vi "Worker Mode Status Example.vi"() -> ()   [LabVIEW 2017]
doc: "------------- lvcsm -------------\n[CSMStates]\nItem 0 = \"Event Structure\"\nItem 1 = \"Idle\"\nItem 2 = \"CSM Documentation\"\nItem 3 = \"VI Reference\"\nItem 4 = \"Error Handler\"\nItem 5 = \"Critical Error\"\nItem 6 = \"Target Busy Error\"\nItem 7 = \"Target Timeout Error\"\nItem 8 = \"Target Error\"\nItem 9 = \"Async Response\"\nItem 10 = \"Response\"\nItem 11 = \"Async Message Posted\"\nItem 12 = \"Initialize Core Data\"\nItem 13 = \"Exit\"\nItem 14 = \"Data: Initialize\"\nItem 15 = \"Data: Cleanup\"\nItem 16 = \"Events: Register\"\nItem 17 = \"Events: Unregister\"\nItem 18 = \"UI: Initialize\"\nItem 19 = \"UI: Cursor Set\"\nItem 20 = \"UI: Front Panel State\"\nItem 21 = \"Macro: Initialize\"\nItem 22 = \"Macro: Switch Active Module\"\nItem 23 = \"Macro: Exit\"\nItem 24 = \"Action: Status Chanage Handler\"\n\n[CSMStatus]"
uses:
  user.lib/_NEVSTOP/Communicable State Machine(CSM)/_Polymophic/Build Synchronous Message with Arguments.vi
  user.lib/_NEVSTOP/Communicable State Machine(CSM)/_Polymophic/Build No-Reply Asynchronous Message with Arguments.vi
  user.lib/_NEVSTOP/Communicable State Machine(CSM)/_Polymophic/Build Unregister Status Message.vi
  user.lib/_NEVSTOP/Communicable State Machine(CSM)/_Polymophic/Build Register Status Message.vi
  user.lib/_NEVSTOP/Communicable State Machine(CSM)/Communicable State Machine.lvlib
  examples/NEVSTOP/Communicable State Machine(CSM)/1. Create a reuse Module/1. Create a reuse Module.lvlib
panel:
  in  "UI: Front Panel State >> Close":bool
  in  "UI: Front Panel State >> Open":bool
  in  "Unregister All Status Change":bool
  in  "API: Stop":bool
  in  "API: Start":bool
  in  "Register All Status Change":bool
  out "State History of Main":string
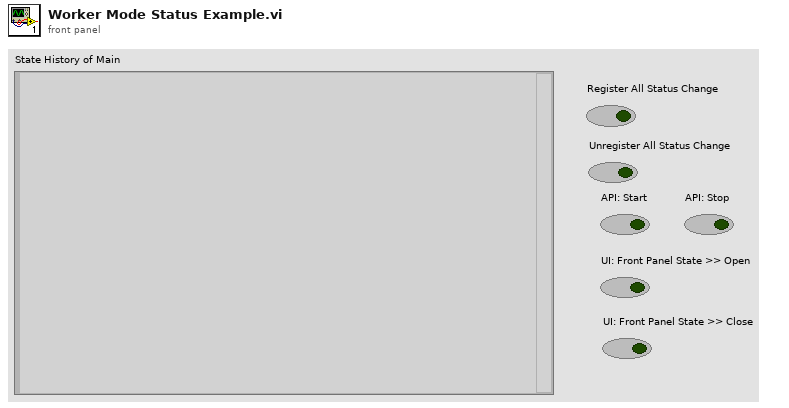
[diagram p1: front panel]
types:
  T1 = enum32{"Invalid", "Standard", "Closed", "Hidden", "Minimized", "Maximized"}
  T2 = enum32{"invalid app kind", "Development System", "Run Time System", "Student Edition", "Embedded LabVIEW", "Evaluation", "Custom"}
  T3 = typedef "Communicable State Machine.lvlib/_CSM_Response Source Message.ctl" = cluster{"‘State":string, "’Arguments":string, "’Error":errorcluster}
  T4 = cluster{"Current VI Reference":refnum<vi>, "Close Panel on Exit?":bool}
  T5 = cluster{"Core":cluster{"Current VI Reference":refnum<vi>, "Close Panel on Exit?":bool}, "Your Boolean data":bool, "Your string data":string}
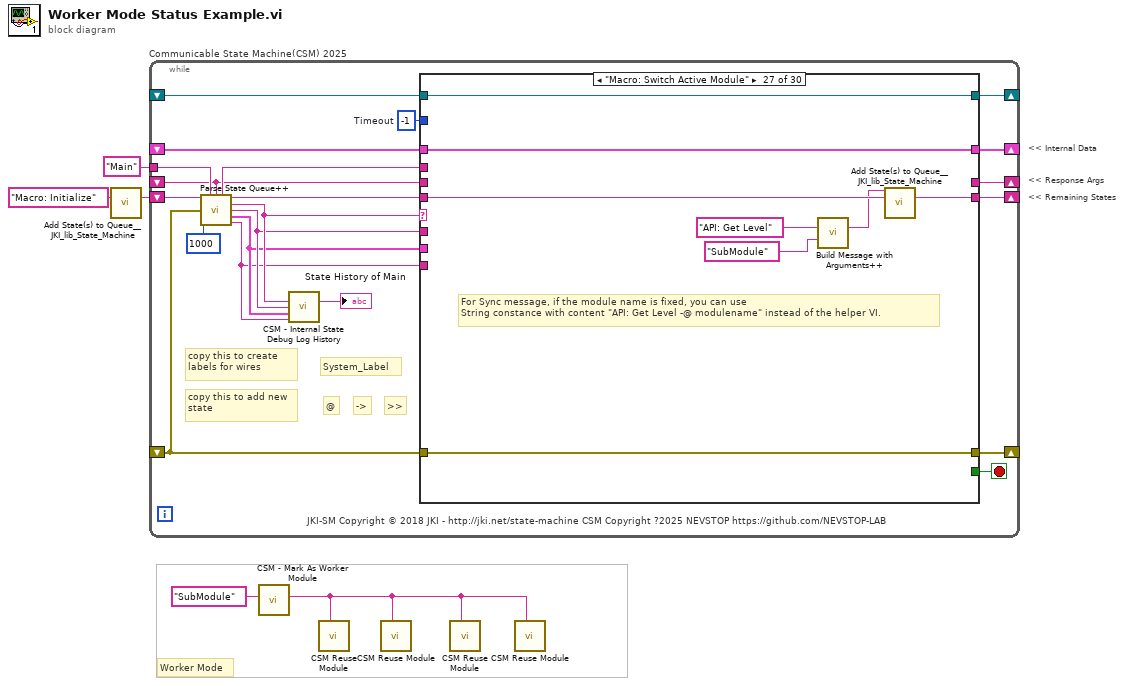
[diagram p0: block diagram]
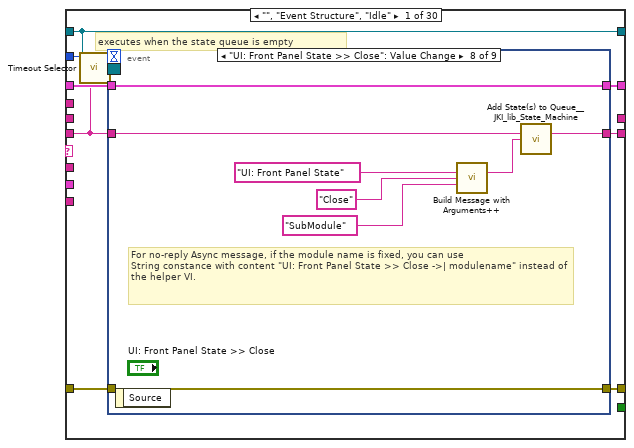
[diagram p2: hidden frame]
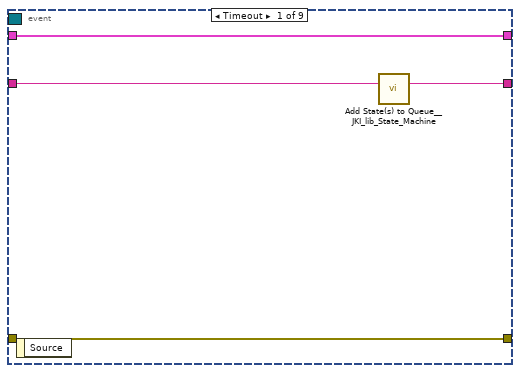
[diagram p3: hidden frame]
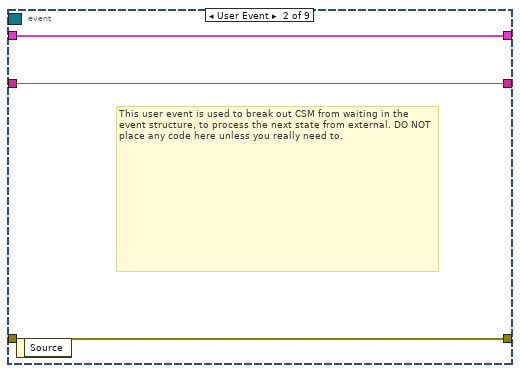
[diagram p4: hidden frame]
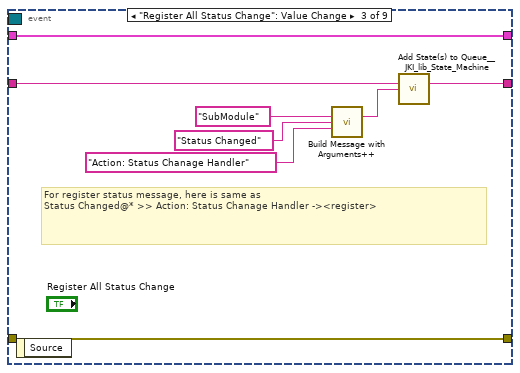
[diagram p5: hidden frame]
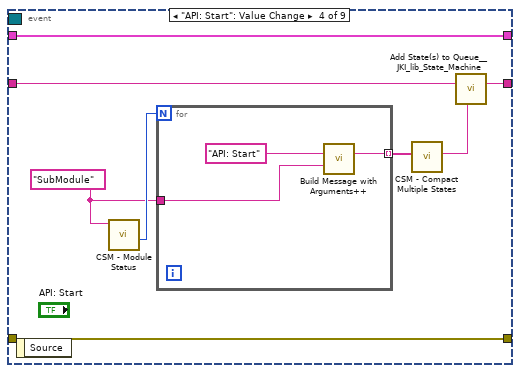
[diagram p6: hidden frame]
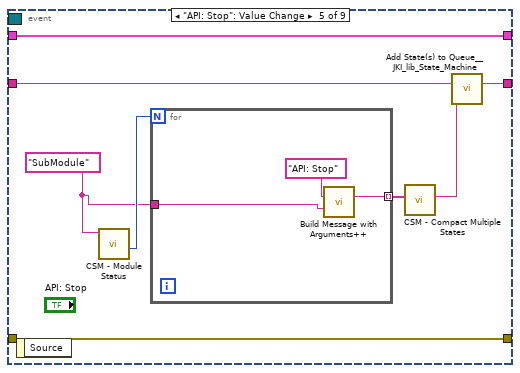
[diagram p7: hidden frame]
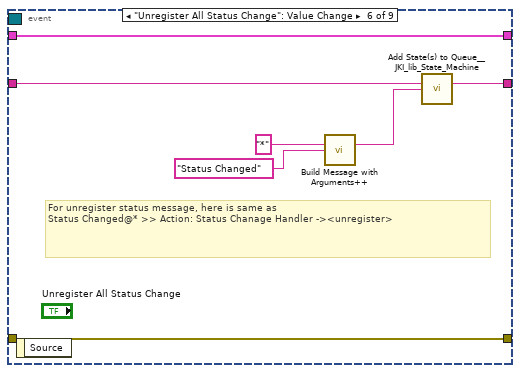
[diagram p8: hidden frame]
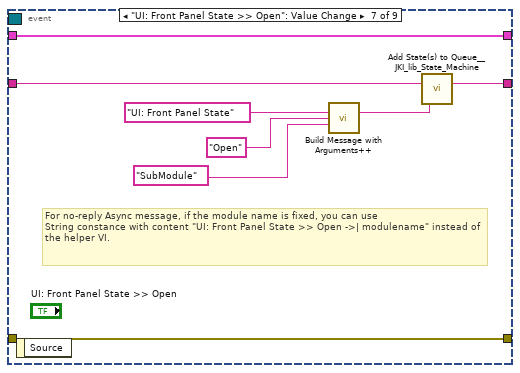
[diagram p9: hidden frame]
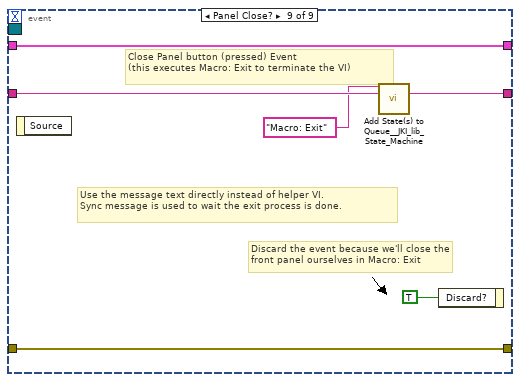
[diagram p10: hidden frame]
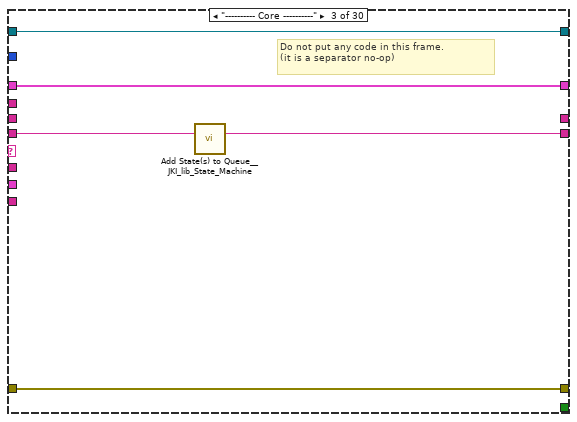
[diagram p12: hidden frame]
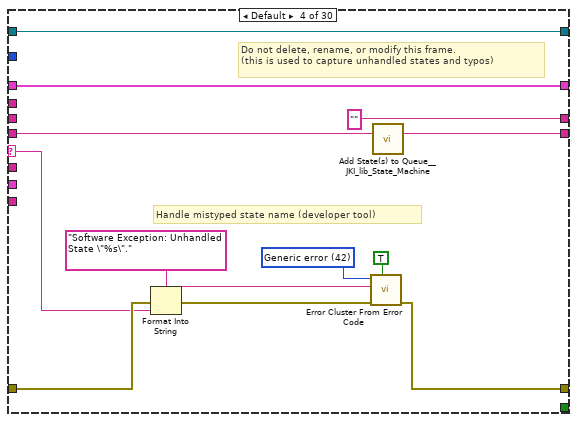
[diagram p13: hidden frame]
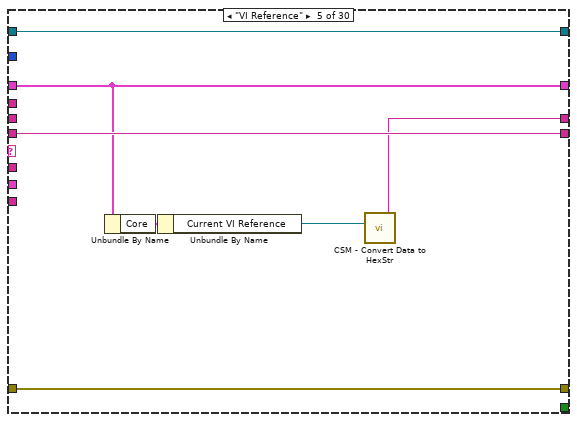
[diagram p14: hidden frame]
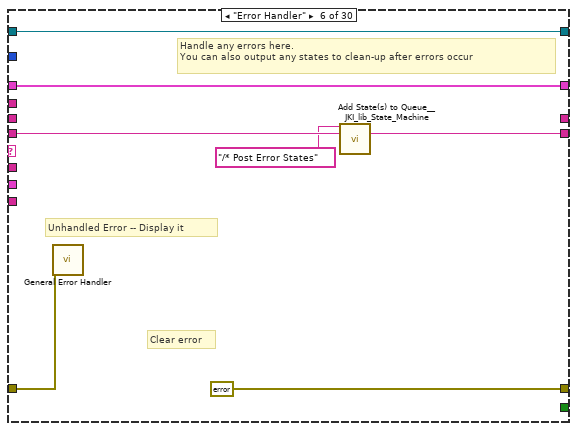
[diagram p15: hidden frame]
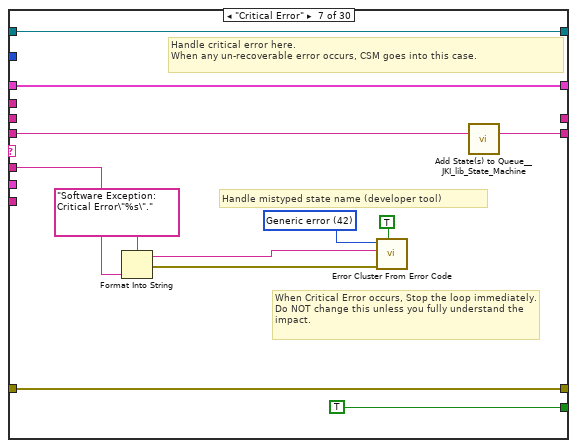
[diagram p16: hidden frame]
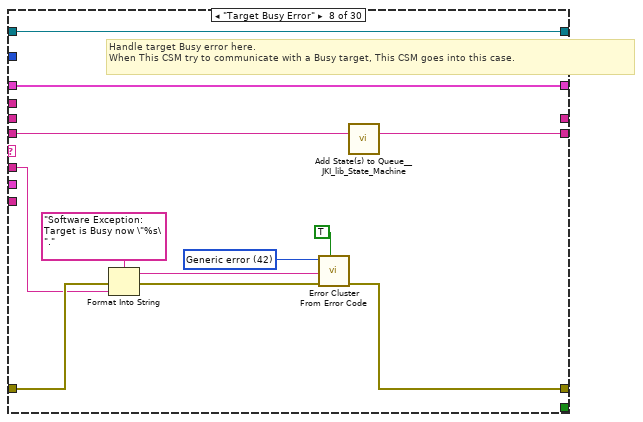
[diagram p17: hidden frame]
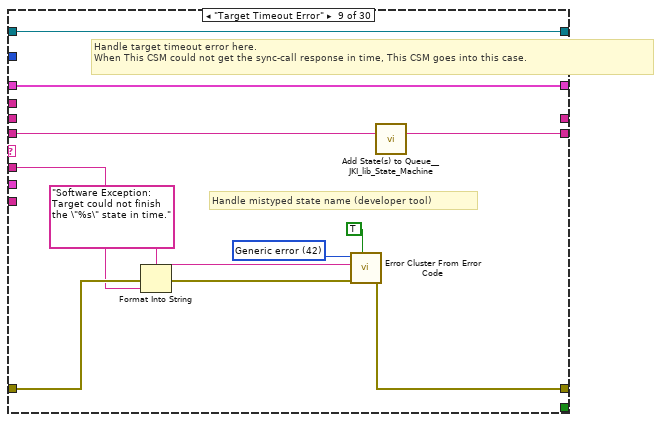
[diagram p18: hidden frame]
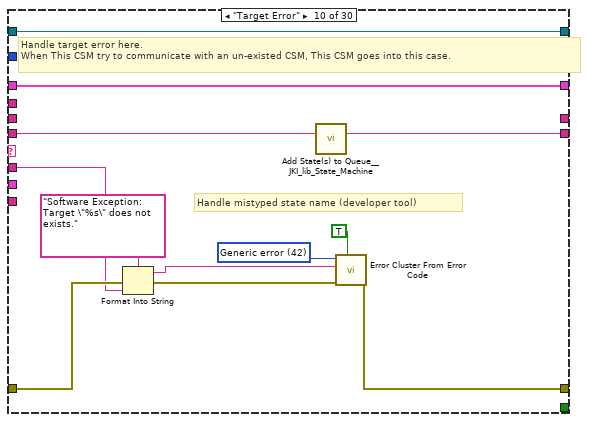
[diagram p19: hidden frame]
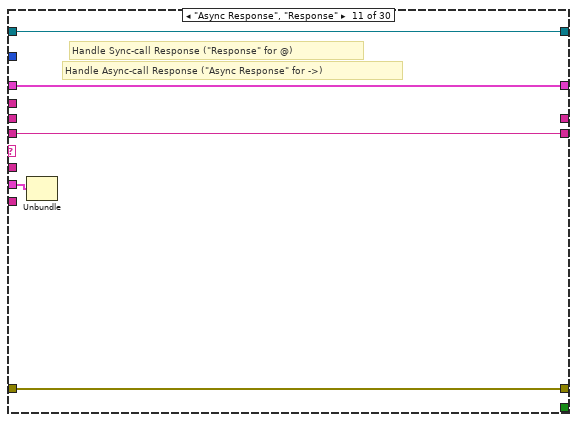
[diagram p20: hidden frame]
diagram:
  # "Worker Mode"
  # "<< Internal Data"
  # "<< Response Args"
  # "<< Remaining States"
  n1 = call <vilib>:"Add State(s) to Queue__JKI_lib_State_Machine.vi"("State(s) in (\"\")"="Macro: Initialize") -> ("States Out"=w5:string)  [unwired: 14 in]
  n2 = while "Communicable State Machine(CSM) 2025" {
    shift-right: [w21] -> _
    shift-left: _ -> [w20]
    shift-right: [w24] -> _
    shift-left: _ -> [w18]
    shift-right: [w23] -> _
    shift-left: w5 -> [w25]
    tunnel: "Main" ("Name(\"\" to use uuid)") -> [w13]
    shift-right: [w16] -> _
    shift-left: _ -> [w7]
    shift-right: [w15] -> _
    shift-left: _ -> [w14]
    stop <- w22 stop-if-true
    w19 = -1  # Timeout
    # "JKI-SM Copyright © 2018 JKI - http://jki.net/state-machine CSM Copyright ?2025 NEVSTOP https://github.com/NEVSTOP-LAB"
    # "copy this to add new state"
    # ">>"
    # "->"
    # "@"
    # "copy this to create labels for wires"
    # "System_Label"
    n3 = call "Parse State Queue++.vi"("State Queue"=w25, "Name (\"\" to Use UUID)"=w13, "Response Arguments"=w7, "Previous Error"=w18, "Response Timeout (-2 Use Global Settings)"=1000 ("Response Timeout(1000ms)")) -> ("Name Used"=w8:string, "Remaining States"=w26:string, "Current State"=w12:string, "Arguments"=w11:string, ">> Response Source Message >>"=w10:T3, ">> Source CSM >>"=w9:string)  [unwired: 5 in]
    n4 = call "CSM - Internal State Debug Log History.vi"("State"=w12, "Arguments (\"\")"=w11, ">> Response Source Message >>"=w10, "Source (\"\")"=w9) -> ("Debug Log"=→"State History of Main":string)  [unwired: 11 in]
    n5 = case shown="\"Macro: Switch Active Module\"" w12 {
      selector: w12 -> [_ _ _ w113 _ _ _ _ _ _ _ _ _ _ _ _ _ _ _ _ _ _ _ _ _ _ _ _ _ _]
      tunnel: w26 -> [w27 w104 w110 w117 w129 w137 w147 w150 w167 w179 w189 w193 w208 w214 w219 w227 w234 w239 w245 w249 w255 w260 w267 w279 w349 w355 w360 w378 w382 w386]
      tunnel: w11 -> [_ _ _ _ _ _ w140 w152 w163 w175 _ _ _ _ _ _ _ _ _ _ _ _ w262 w273 _ _ _ _ _ _]
      tunnel: w20 -> [w34 w103 w107 w115 w128 w134 w148 w154 w165 w177 w188 w192 w201 w212 w216 _ w229 w236 w244 w248 w252 w256 w265 w275 w346 w352 w358 w375 w381 w385]
      tunnel: [w33 w105 w108 w119 w130 errorcluster {"status"=FALSE, "code"=0, "source"=""} ("error out") w149 w157 w169 w181 w190 w194 w205 w211 w217 w224 w230 w237 w240 w247 w253 w258 w263 w276 w347 w353 w363 w376 w383 w387] -> w24
      tunnel: w18 -> [w32 w105 w108 w118 w130 w133 w149 w156 w168 w180 w190 w194 w205 w211 w217 w224 w231 w237 _ w250 w253 w258 w264 w277 w347 w353 w363 w376 w383 w387]
      tunnel: [w35 w104 w109 w116 w129 w136 w146 w155 w166 w178 w189 w193 w207 w213 w218 w226 w233 w238 w245 w249 w254 w259 w266 w278 w348 w354 w361 w377 w382 w386] -> w23
      tunnel: [_ _ _ _ _ _ TRUE _ _ _ _ _ _ TRUE _ _ _ _ _ _ _ _ _ _ _ _ _ _ _ _] -> w22
      tunnel: [w31 w103 w107 w115 w128 w134 w148 w154 w165 w177 w188 w192 w206 w212 w216 w225 w229 w236 w244 w248 w252 w256 w265 w275 w346 w352 w358 w375 w381 w385] -> w21
      tunnel: w19 -> [w30 _ _ _ _ _ _ _ _ _ _ _ _ _ _ _ _ _ _ _ _ _ _ _ _ _ _ _ _ _]
      tunnel: w9 -> [_ _ _ _ _ _ _ _ _ _ _ _ _ _ _ _ _ _ _ _ _ _ _ _ _ _ _ _ _ _]
      tunnel: w10 -> [_ _ _ _ _ _ _ _ _ _ w186 _ _ _ _ _ _ _ _ _ _ _ _ _ _ _ _ _ _ _]
      tunnel: [_ _ _ "" w124 _ _ _ _ _ _ _ _ _ _ _ _ _ _ _ _ _ _ _ _ _ _ _ _ _] -> w16
      tunnel: [w29 w102 w106 w111 w127 w131 w138 w151 w162 w174 w187 w191 w195 w209 w215 w220 w228 w235 w243 w246 w251 w257 w261 w272 w345 w350 w362 w368 w380 w384] -> w15
      tunnel: w14 -> [w29 w102 w106 w111 w127 w131 w138 w151 w162 w174 w187 w191 w195 w209 w215 w220 w228 w235 _ w246 w251 w257 w261 w272 w345 w350 w362 w368 w380 w384]
      tunnel: w8 -> [_ _ _ _ _ _ _ _ _ _ _ _ _ _ _ _ _ _ w242 _ _ _ _ _ _ _ _ _ _ _]
      tunnel: w7 -> [_ _ _ _ _ _ _ _ _ _ _ _ _ _ _ _ _ _ _ _ _ _ _ _ _ _ _ _ _ _]
      frame "", "Event Structure", "Idle" {
        # "executes when the state queue is empty"
        n6 = call "Timeout Selector.vi"("Remaining States"=w27, "Timeout Expected"=w30) -> ("Timeout"=w28:i32)  [unwired: 5 in]
        n7 = event shown="[7] \"UI: Front Panel State >> Close\": Value Change" {
          selector: w29 -> [_ _ _ _ _ _ _ _ _]
          dyn-events: _ -> [_ _ _ _ _ _ _ _ _]
          timeout: w28 -> [_ _ _ _ _ _ _ _ _]
          tunnel: w27 -> [w39 w41 w48 w57 w68 w77 w86 w94 w101]
          tunnel: [w38 w41 w47 w56 w67 w76 w85 w93 w100] -> w35
          tunnel: w34 -> [w36 w42 w49 w54 w65 w78 w84 w91 w98]
          tunnel: [w37 w40 w50 w58 w69 w79 w87 w95 w99] -> w33
          tunnel: w32 -> [w37 w40 w50 w58 w69 w79 w87 w95 w99]
          tunnel: [w36 w42 w49 w54 w65 w78 w84 w91 w98] -> w31
          event Timeout {
            n8 = event-data() -> ()  [unwired: 1 in, 1 out]
            n9 = call <vilib>:"Add State(s) to Queue__JKI_lib_State_Machine.vi"("State(s) in (\"\")"=w39) -> ("States Out"=w38:string)  [unwired: 14 in]
          }
          event User Event {
            # "This user event is used to break out CSM from waiting in the event structure, to process the next state from external. DO NOT place any code here unless you really need to."
            n10 = event-data() -> ()  [unwired: 1 in, 1 out]
          }
          event "Register All Status Change": Value Change {
            # "For register status message, here is same as \nStatus Changed@* >> Action: Status Chanage Handler -><register>"
            n11 = event-data() -> ()  [unwired: 1 in, 1 out]
            n12 = call-poly "Build Message with Arguments++.vi"("Source CSM (* as Default)"="SubModule" ("Source CSM Name (* as Default)"), "Status"="Status Changed", "API (If \"\", Same As \"Status\")"="Action: Status Chanage Handler" ("Status")) -> ("CSM Message String"=w43:string)  [unwired: 12 in]
            n13 = call <vilib>:"Add State(s) to Queue__JKI_lib_State_Machine.vi"("State(s) in (\"\")"=w48, "State(s) at Back (\"\")"=w43) -> ("States Out"=w47:string)  [unwired: 13 in]
          }
          event "API: Start": Value Change {
            w51 = "SubModule" ("CSM Name")
            n14 = event-data() -> ()  [unwired: 1 in, 1 out]
            n15 = call "CSM - Module Status.vi"("CSM Name"=w51) -> ("#Instance"=w53:i32)  [unwired: 6 in, 4 out]
            n16 = for {
              N: w53 -> [_]
              tunnel: [w60] -> w55 mode=indexing
              tunnel: w51 -> [w59]
              n17 = call-poly "Build Message with Arguments++.vi"("State With Arguments"="API: Start" ("State(s) in Front (\"\")"), "Target Module (\"\")"=w59) -> ("CSM Message String"=w60:string)  [unwired: 13 in]
            }
            n18 = call "CSM - Compact Multiple States.vi"("Multiple States"=w55) -> ("States"=w52:string)  [unwired: 9 in]
            n19 = call <vilib>:"Add State(s) to Queue__JKI_lib_State_Machine.vi"("State(s) in (\"\")"=w57, "State(s) at Back (\"\")"=w52) -> ("States Out"=w56:string)  [unwired: 13 in]
          }
          event "API: Stop": Value Change {
            w62 = "SubModule" ("CSM Name")
            n20 = event-data() -> ()  [unwired: 1 in, 1 out]
            n21 = call "CSM - Module Status.vi"("CSM Name"=w62) -> ("#Instance"=w64:i32)  [unwired: 6 in, 4 out]
            n22 = for {
              N: w64 -> [_]
              tunnel: [w71] -> w66 mode=indexing
              tunnel: w62 -> [w70]
              n23 = call-poly "Build Message with Arguments++.vi"("State With Arguments"="API: Stop" ("State(s) in Front (\"\")"), "Target Module (\"\")"=w70) -> ("CSM Message String"=w71:string)  [unwired: 13 in]
            }
            n24 = call "CSM - Compact Multiple States.vi"("Multiple States"=w66) -> ("States"=w63:string)  [unwired: 9 in]
            n25 = call <vilib>:"Add State(s) to Queue__JKI_lib_State_Machine.vi"("State(s) in (\"\")"=w68, "State(s) at Back (\"\")"=w63) -> ("States Out"=w67:string)  [unwired: 13 in]
          }
          event "Unregister All Status Change": Value Change {
            # "For unregister status message, here is same as \nStatus Changed@* >> Action: Status Chanage Handler -><unregister>"
            n26 = event-data() -> ()  [unwired: 1 in, 1 out]
            n27 = call-poly "Build Message with Arguments++.vi"("Source CSM (* as Default)"="*" ("Source CSM Name (* as Default)"), "Status"="Status Changed") -> ("CSM Message String"=w73:string)  [unwired: 13 in]
            n28 = call <vilib>:"Add State(s) to Queue__JKI_lib_State_Machine.vi"("State(s) in (\"\")"=w77, "State(s) at Back (\"\")"=w73) -> ("States Out"=w76:string)  [unwired: 13 in]
          }
          event "UI: Front Panel State >> Open": Value Change {
            # "For no-reply Async message, if the module name is fixed, you can use\nString constance with content \"UI: Front Panel State >> Open ->| modulename\" instead of the helper VI."
            n29 = event-data() -> ()  [unwired: 1 in, 1 out]
            n30 = call-poly "Build Message with Arguments++.vi"("State With Arguments"="UI: Front Panel State" ("CSM Name"), "Arguments (\"\")"="Open" ("CSM Name"), "Target Module (\"\")"="SubModule" ("Name(\"\" to use uuid)")) -> ("CSM Message String"=w83:string)  [unwired: 12 in]
            n31 = call <vilib>:"Add State(s) to Queue__JKI_lib_State_Machine.vi"("State(s) in (\"\")"=w86, "State(s) at Back (\"\")"=w83) -> ("States Out"=w85:string)  [unwired: 13 in]
          }
          event "UI: Front Panel State >> Close": Value Change {
            # "For no-reply Async message, if the module name is fixed, you can use\nString constance with content \"UI: Front Panel State >> Close ->| modulename\" instead of the helper VI."
            n32 = event-data() -> ()  [unwired: 1 in, 1 out]
            n33 = call-poly "Build Message with Arguments++.vi"("State With Arguments"="UI: Front Panel State" ("CSM Name"), "Arguments (\"\")"="Close" ("CSM Name"), "Target Module (\"\")"="SubModule" ("Name(\"\" to use uuid)")) -> ("CSM Message String"=w90:string)  [unwired: 12 in]
            n34 = call <vilib>:"Add State(s) to Queue__JKI_lib_State_Machine.vi"("State(s) in (\"\")"=w94, "State(s) at Back (\"\")"=w90) -> ("States Out"=w93:string)  [unwired: 13 in]
          }
          event Panel Close? {
            # "Use the message text directly instead of helper VI.\nSync message is used to wait the exit process is done."
            # "Discard the event because we'll close the front panel ourselves in Macro: Exit"
            # "Close Panel button (pressed) Event\n(this executes Macro: Exit to terminate the VI)"
            n35 = event-data() -> ()  [unwired: 1 in, 1 out]
            n36 = call <vilib>:"Add State(s) to Queue__JKI_lib_State_Machine.vi"("State(s) in Front (\"\")"="Macro: Exit", "State(s) in (\"\")"=w101) -> ("States Out"=w100:string)  [unwired: 13 in]
            n37 = event-data("Discard?"=TRUE) -> ()  [unwired: 1 in, 1 out]
          }
        }
      }
      frame "CSM Documentation" {
        # "#CSM README FIRST\n\nCSM is a LabVIEW application framework that builds upon JKI State Machine (JKISM). It follows the pattern of JKISM and extends the keywords to describe message communication between CSM modules, including concepts such as Sync-Message, Async-Message, Subscription/Unsubscription of status - essential elements for creating reusable code modules. For more information, please visit the CSM wiki: https://github.com/NEVSTOP-LAB/JKI-State-Machine-Plus-Plus/wiki\n\nFor instructions on JKI State Machine, visit: http://jki.net/state-machine/\nFor information about CSM, visit: https://github.com/NEVSTOP-LAB"
        # "CSM Documentation"
      }
      frame "---------- Core ----------" {
        # "Do not put any code in this frame.\n(it is a separator no-op)"
        n38 = call <vilib>:"Add State(s) to Queue__JKI_lib_State_Machine.vi"("State(s) in (\"\")"=w110) -> ("States Out"=w109:string)  [unwired: 14 in]
      }
      frame Default {
        w122 = 42 items=["No error", "Argument error", "Memory is full", "Out of zone", "End of file", "File already open", "Generic file I/O error", "File not found", "File permission error", "Disk is full", "Duplicate path", "Too many files open", "System feature not enabled", "Resource file not found", "Cannot add resource", "Resource not found", "Image not found", "Image memory error", "Pen does not exist", "Config type invalid", "Config token not found", "Config parse error", "Config memory error", "Bad external code format", "Bad external code offset", "External code not present", "Null window", "Destroy window error", "Null menu", "Print aborted", "Bad print record", "Print driver error", "Windows error during printing", "Memory error during printing", "Print dialog error", "Generic print error", "Invalid device refnum", "Device not found", "Device parameter error", "Device unit error", "Cannot open device", "Device call aborted", "Generic error", "Cancelled by user", "Object ID too low", "Object ID too high", "Object not in heap", "Unknown heap", "Unknown object (invalid DefProc)", "Unknown object (DefProc not in table)", "Message out of range", "Invalid (null) method", "Unknown message", "Manager call not supported", "Bad address", "Network operation in progress", "Network operation timed out", "Connection is busy", "Network attribute not supported", "Network error", "Address in use", "System out of memory", "Connection aborted", "Connection refused", "Not connected", "Already connected", "Connection closed", "Initialization error (interapplication manager)", "Bad occurrence", "Wait on unbound occurrence handler", "Occurrence queue overflow", "Datalog type conflict", "Unused", "Unrecognized type (interapplication manager)", "Memory corrupt", "Failed to make temporary DLL", "Old CIN version", "Drag socket not found", "Failed to load drop-object", "Failed to register OLE object", "Failed to release OLE object", "Format specifier type mismatch", "Unknown format specifier", "Too few format specifiers", "Too many format specifiers", "Scan failed", "Newer CIN version", "Error converting to variant", "Runtime menu error", "Password tampered", "Variant attribute not found", "Incompatible variant data type", "Event data is not available", "Event Store is not present", "Occurrence is not found", "Event Queue is not created", "Event info is not available", "Refnum passed is NULL", "Error retrieving Class GUID", "Error retrieving CoClass GUID", "Error retrieving TypeLib GUID.", "Bad built application magic bytes.", "Specific driver is different from the specific driver associated with the Logical Name.", "There is no session opened to the class driver.", "Max Error", "MAX - Error with config objects", "MAX - Error loading configuration", "MAX - Group not supported"]
        # "Do not delete, rename, or modify this frame.\n(this is used to capture unhandled states and typos)"
        # "Handle mistyped state name (developer tool)"
        n39 = Format Into String(format string="Software Exception: Unhandled State \"%s\"." ("message"), error in=w118, w113) -> (resulting string=w121:string, error out=w120:errorcluster)  [unwired: 1 in]
        n40 = call <vilib>:"Error Cluster From Error Code.vi"("show call chain? (False)"=TRUE, "error in (no error)"=w120, "error message (\"\")"=w121, "error code (0)"=w122) -> ("error out"=w119:errorcluster)  [unwired: 5 in]
        n41 = call <vilib>:"Add State(s) to Queue__JKI_lib_State_Machine.vi"("State(s) in (\"\")"=w117) -> ("States Out"=w116:string)  [unwired: 14 in]
      }
      frame "VI Reference" {
        n42 = Unbundle By Name(w128) -> ("Core"=w126:T4)
        n43 = Unbundle By Name(w126) -> ("Current VI Reference"=w125:refnum<vi>)
        n44 = call "CSM - Convert Data to HexStr.vi"("Variant"=w125) -> ("HEX String (0-9,A-F)"=w124:string)  [unwired: 8 in]
      }
      frame "Error Handler" {
        # "Unhandled Error -- Display it"
        # "Handle any errors here.\nYou can also output any states to clean-up after errors occur"
        # "Clear error"
        n45 = call <vilib>:"General Error Handler.vi"("error in (no error)"=w133) -> ()  [unwired: 10 in, 5 out]
        n46 = call <vilib>:"Add State(s) to Queue__JKI_lib_State_Machine.vi"("State(s) in Front (\"\")"="/* Post Error States", "State(s) in (\"\")"=w137) -> ("States Out"=w136:string)  [unwired: 13 in]
      }
      frame "Critical Error" {
        w144 = 42 items=["No error", "Argument error", "Memory is full", "Out of zone", "End of file", "File already open", "Generic file I/O error", "File not found", "File permission error", "Disk is full", "Duplicate path", "Too many files open", "System feature not enabled", "Resource file not found", "Cannot add resource", "Resource not found", "Image not found", "Image memory error", "Pen does not exist", "Config type invalid", "Config token not found", "Config parse error", "Config memory error", "Bad external code format", "Bad external code offset", "External code not present", "Null window", "Destroy window error", "Null menu", "Print aborted", "Bad print record", "Print driver error", "Windows error during printing", "Memory error during printing", "Print dialog error", "Generic print error", "Invalid device refnum", "Device not found", "Device parameter error", "Device unit error", "Cannot open device", "Device call aborted", "Generic error", "Cancelled by user", "Object ID too low", "Object ID too high", "Object not in heap", "Unknown heap", "Unknown object (invalid DefProc)", "Unknown object (DefProc not in table)", "Message out of range", "Invalid (null) method", "Unknown message", "Manager call not supported", "Bad address", "Network operation in progress", "Network operation timed out", "Connection is busy", "Network attribute not supported", "Network error", "Address in use", "System out of memory", "Connection aborted", "Connection refused", "Not connected", "Already connected", "Connection closed", "Initialization error (interapplication manager)", "Bad occurrence", "Wait on unbound occurrence handler", "Occurrence queue overflow", "Datalog type conflict", "Unused", "Unrecognized type (interapplication manager)", "Memory corrupt", "Failed to make temporary DLL", "Old CIN version", "Drag socket not found", "Failed to load drop-object", "Failed to register OLE object", "Failed to release OLE object", "Format specifier type mismatch", "Unknown format specifier", "Too few format specifiers", "Too many format specifiers", "Scan failed", "Newer CIN version", "Error converting to variant", "Runtime menu error", "Password tampered", "Variant attribute not found", "Incompatible variant data type", "Event data is not available", "Event Store is not present", "Occurrence is not found", "Event Queue is not created", "Event info is not available", "Refnum passed is NULL", "Error retrieving Class GUID", "Error retrieving CoClass GUID", "Error retrieving TypeLib GUID.", "Bad built application magic bytes.", "Specific driver is different from the specific driver associated with the Logical Name.", "There is no session opened to the class driver.", "Max Error", "MAX - Error with config objects", "MAX - Error loading configuration", "MAX - Group not supported"]
        # "Handle critical error here.\nWhen any un-recoverable error occurs, CSM goes into this case."
        # "When Critical Error occurs, Stop the loop immediately. Do NOT change this unless you fully understand the impact."
        # "Handle mistyped state name (developer tool)"
        n47 = Format Into String(format string="Software Exception: Critical Error\"%s\"." ("message"), w140) -> (resulting string=w143:string, error out=w142:errorcluster)  [unwired: 2 in]
        n48 = call <vilib>:"Error Cluster From Error Code.vi"("show call chain? (False)"=TRUE, "error in (no error)"=w142, "error message (\"\")"=w143, "error code (0)"=w144) -> ()  [unwired: 5 in, 1 out]
        n49 = call <vilib>:"Add State(s) to Queue__JKI_lib_State_Machine.vi"("State(s) in (\"\")"=w147) -> ("States Out"=w146:string)  [unwired: 14 in]
      }
      frame "Target Busy Error" {
        w160 = 42 items=["No error", "Argument error", "Memory is full", "Out of zone", "End of file", "File already open", "Generic file I/O error", "File not found", "File permission error", "Disk is full", "Duplicate path", "Too many files open", "System feature not enabled", "Resource file not found", "Cannot add resource", "Resource not found", "Image not found", "Image memory error", "Pen does not exist", "Config type invalid", "Config token not found", "Config parse error", "Config memory error", "Bad external code format", "Bad external code offset", "External code not present", "Null window", "Destroy window error", "Null menu", "Print aborted", "Bad print record", "Print driver error", "Windows error during printing", "Memory error during printing", "Print dialog error", "Generic print error", "Invalid device refnum", "Device not found", "Device parameter error", "Device unit error", "Cannot open device", "Device call aborted", "Generic error", "Cancelled by user", "Object ID too low", "Object ID too high", "Object not in heap", "Unknown heap", "Unknown object (invalid DefProc)", "Unknown object (DefProc not in table)", "Message out of range", "Invalid (null) method", "Unknown message", "Manager call not supported", "Bad address", "Network operation in progress", "Network operation timed out", "Connection is busy", "Network attribute not supported", "Network error", "Address in use", "System out of memory", "Connection aborted", "Connection refused", "Not connected", "Already connected", "Connection closed", "Initialization error (interapplication manager)", "Bad occurrence", "Wait on unbound occurrence handler", "Occurrence queue overflow", "Datalog type conflict", "Unused", "Unrecognized type (interapplication manager)", "Memory corrupt", "Failed to make temporary DLL", "Old CIN version", "Drag socket not found", "Failed to load drop-object", "Failed to register OLE object", "Failed to release OLE object", "Format specifier type mismatch", "Unknown format specifier", "Too few format specifiers", "Too many format specifiers", "Scan failed", "Newer CIN version", "Error converting to variant", "Runtime menu error", "Password tampered", "Variant attribute not found", "Incompatible variant data type", "Event data is not available", "Event Store is not present", "Occurrence is not found", "Event Queue is not created", "Event info is not available", "Refnum passed is NULL", "Error retrieving Class GUID", "Error retrieving CoClass GUID", "Error retrieving TypeLib GUID.", "Bad built application magic bytes.", "Specific driver is different from the specific driver associated with the Logical Name.", "There is no session opened to the class driver.", "Max Error", "MAX - Error with config objects", "MAX - Error loading configuration", "MAX - Group not supported"]
        # "Handle target Busy error here.\nWhen This CSM try to communicate with a Busy target, This CSM goes into this case."
        n50 = Format Into String(format string="Software Exception: Target is Busy now \"%s\"." ("message"), error in=w156, w152) -> (resulting string=w159:string, error out=w158:errorcluster)  [unwired: 1 in]
        n51 = call <vilib>:"Error Cluster From Error Code.vi"("show call chain? (False)"=TRUE, "error in (no error)"=w158, "error message (\"\")"=w159, "error code (0)"=w160) -> ("error out"=w157:errorcluster)  [unwired: 5 in]
        n52 = call <vilib>:"Add State(s) to Queue__JKI_lib_State_Machine.vi"("State(s) in (\"\")"=w150) -> ("States Out"=w155:string)  [unwired: 14 in]
      }
      frame "Target Timeout Error" {
        w172 = 42 items=["No error", "Argument error", "Memory is full", "Out of zone", "End of file", "File already open", "Generic file I/O error", "File not found", "File permission error", "Disk is full", "Duplicate path", "Too many files open", "System feature not enabled", "Resource file not found", "Cannot add resource", "Resource not found", "Image not found", "Image memory error", "Pen does not exist", "Config type invalid", "Config token not found", "Config parse error", "Config memory error", "Bad external code format", "Bad external code offset", "External code not present", "Null window", "Destroy window error", "Null menu", "Print aborted", "Bad print record", "Print driver error", "Windows error during printing", "Memory error during printing", "Print dialog error", "Generic print error", "Invalid device refnum", "Device not found", "Device parameter error", "Device unit error", "Cannot open device", "Device call aborted", "Generic error", "Cancelled by user", "Object ID too low", "Object ID too high", "Object not in heap", "Unknown heap", "Unknown object (invalid DefProc)", "Unknown object (DefProc not in table)", "Message out of range", "Invalid (null) method", "Unknown message", "Manager call not supported", "Bad address", "Network operation in progress", "Network operation timed out", "Connection is busy", "Network attribute not supported", "Network error", "Address in use", "System out of memory", "Connection aborted", "Connection refused", "Not connected", "Already connected", "Connection closed", "Initialization error (interapplication manager)", "Bad occurrence", "Wait on unbound occurrence handler", "Occurrence queue overflow", "Datalog type conflict", "Unused", "Unrecognized type (interapplication manager)", "Memory corrupt", "Failed to make temporary DLL", "Old CIN version", "Drag socket not found", "Failed to load drop-object", "Failed to register OLE object", "Failed to release OLE object", "Format specifier type mismatch", "Unknown format specifier", "Too few format specifiers", "Too many format specifiers", "Scan failed", "Newer CIN version", "Error converting to variant", "Runtime menu error", "Password tampered", "Variant attribute not found", "Incompatible variant data type", "Event data is not available", "Event Store is not present", "Occurrence is not found", "Event Queue is not created", "Event info is not available", "Refnum passed is NULL", "Error retrieving Class GUID", "Error retrieving CoClass GUID", "Error retrieving TypeLib GUID.", "Bad built application magic bytes.", "Specific driver is different from the specific driver associated with the Logical Name.", "There is no session opened to the class driver.", "Max Error", "MAX - Error with config objects", "MAX - Error loading configuration", "MAX - Group not supported"]
        # "Handle target timeout error here.\nWhen This CSM could not get the sync-call response in time, This CSM goes into this case."
        # "Handle mistyped state name (developer tool)"
        n53 = Format Into String(format string="Software Exception: Target could not finish the \"%s\" state in time." ("message"), error in=w168, w163) -> (resulting string=w171:string, error out=w170:errorcluster)  [unwired: 1 in]
        n54 = call <vilib>:"Error Cluster From Error Code.vi"("show call chain? (False)"=TRUE, "error in (no error)"=w170, "error message (\"\")"=w171, "error code (0)"=w172) -> ("error out"=w169:errorcluster)  [unwired: 5 in]
        n55 = call <vilib>:"Add State(s) to Queue__JKI_lib_State_Machine.vi"("State(s) in (\"\")"=w167) -> ("States Out"=w166:string)  [unwired: 14 in]
      }
      frame "Target Error" {
        w184 = 42 items=["No error", "Argument error", "Memory is full", "Out of zone", "End of file", "File already open", "Generic file I/O error", "File not found", "File permission error", "Disk is full", "Duplicate path", "Too many files open", "System feature not enabled", "Resource file not found", "Cannot add resource", "Resource not found", "Image not found", "Image memory error", "Pen does not exist", "Config type invalid", "Config token not found", "Config parse error", "Config memory error", "Bad external code format", "Bad external code offset", "External code not present", "Null window", "Destroy window error", "Null menu", "Print aborted", "Bad print record", "Print driver error", "Windows error during printing", "Memory error during printing", "Print dialog error", "Generic print error", "Invalid device refnum", "Device not found", "Device parameter error", "Device unit error", "Cannot open device", "Device call aborted", "Generic error", "Cancelled by user", "Object ID too low", "Object ID too high", "Object not in heap", "Unknown heap", "Unknown object (invalid DefProc)", "Unknown object (DefProc not in table)", "Message out of range", "Invalid (null) method", "Unknown message", "Manager call not supported", "Bad address", "Network operation in progress", "Network operation timed out", "Connection is busy", "Network attribute not supported", "Network error", "Address in use", "System out of memory", "Connection aborted", "Connection refused", "Not connected", "Already connected", "Connection closed", "Initialization error (interapplication manager)", "Bad occurrence", "Wait on unbound occurrence handler", "Occurrence queue overflow", "Datalog type conflict", "Unused", "Unrecognized type (interapplication manager)", "Memory corrupt", "Failed to make temporary DLL", "Old CIN version", "Drag socket not found", "Failed to load drop-object", "Failed to register OLE object", "Failed to release OLE object", "Format specifier type mismatch", "Unknown format specifier", "Too few format specifiers", "Too many format specifiers", "Scan failed", "Newer CIN version", "Error converting to variant", "Runtime menu error", "Password tampered", "Variant attribute not found", "Incompatible variant data type", "Event data is not available", "Event Store is not present", "Occurrence is not found", "Event Queue is not created", "Event info is not available", "Refnum passed is NULL", "Error retrieving Class GUID", "Error retrieving CoClass GUID", "Error retrieving TypeLib GUID.", "Bad built application magic bytes.", "Specific driver is different from the specific driver associated with the Logical Name.", "There is no session opened to the class driver.", "Max Error", "MAX - Error with config objects", "MAX - Error loading configuration", "MAX - Group not supported"]
        # "Handle target error here.\nWhen This CSM try to communicate with an un-existed CSM, This CSM goes into this case."
        # "Handle mistyped state name (developer tool)"
        n56 = Format Into String(format string="Software Exception: Target \"%s\" does not exists." ("message"), error in=w180, w175) -> (resulting string=w183:string, error out=w182:errorcluster)  [unwired: 1 in]
        n57 = call <vilib>:"Add State(s) to Queue__JKI_lib_State_Machine.vi"("State(s) in (\"\")"=w179) -> ("States Out"=w178:string)  [unwired: 14 in]
        n58 = call <vilib>:"Error Cluster From Error Code.vi"("show call chain? (False)"=TRUE, "error in (no error)"=w182, "error message (\"\")"=w183, "error code (0)"=w184) -> ("error out"=w181:errorcluster)  [unwired: 5 in]
      }
      frame "Async Response", "Response" {
        # "Handle Async-call Response (\"Async Response\" for ->)"
        # "Handle Sync-call Response (\"Response\" for @)"
        n59 = Unbundle(w186) -> ()  [unwired: 3 out]
      }
      frame "Async Message Posted" {
        # "Handle post action for async message (->)."
        # "After Async Message is posted (->), CSM goes to this state for post-action. You can use Argument - State to tell which Async Message is called."
      }
      frame "Initialize Core Data" {
        # "Do not delete, rename, or modify this frame.\n(this is used to determine panel behavior on exit)"
        # "originally closed?"
        # "exe?"
        # "If panel starts closed or is an EXE, then close it when we exit"
        n60 = property class="VI"() -> ("FP.State"=w198:T1)  [unwired: 2 in, 2 out]
        n61 = property class="App"() -> ("App.Kind"=w204:T2)  [unwired: 2 in, 2 out]
        n62 = control-ref of="Current VI Reference"() -> (w199:refnum<vi>)
        n63 = Equal?(x=w198, y=T1."Closed" ("Front Panel Window:State")) -> (x = y?=w196:bool)
        n64 = Equal?(x=w204, y=T2."Run Time System" ("Application:Kind")) -> (x = y?=w202:bool)
        n65 = Or(x=w196, y=w202) -> (x .or. y?=w200:bool)
        n66 = Bundle By Name(cluster=w201, "Core.Current VI Reference"=w199, "Core.Close Panel on Exit?"=w200) -> (w206:T5)
        n67 = call <vilib>:"Add State(s) to Queue__JKI_lib_State_Machine.vi"("State(s) in (\"\")"=w208) -> ("States Out"=w207:string)  [unwired: 14 in]
      }
      frame "Exit" {
        # "Do not put any code in this frame.\n(No errors that occur here will be handled.)"
        n68 = call <vilib>:"Add State(s) to Queue__JKI_lib_State_Machine.vi"("State(s) in (\"\")"=w214) -> ("States Out"=w213:string)  [unwired: 14 in]
      }
      frame "---------- Data ----------" {
        # "Do not put any code in this frame.\n(It is a separator no-op. You can make a copy of this frame to create a new Data frame)"
        n69 = call <vilib>:"Add State(s) to Queue__JKI_lib_State_Machine.vi"("State(s) in (\"\")"=w219) -> ("States Out"=w218:string)  [unwired: 14 in]
      }
      frame "Data: Initialize" {
        w221 = T4 {"Current VI Reference"=refnum, "Close Panel on Exit?"=FALSE}  # Core
        w223 = TRUE  # Your Boolean data
        w222 = ""  # Your string data
        # "do not delete - used by framework"
        # "Initialize the shift-register data, here.\n(data names are defined by what you wire into the bundle function)"
        n70 = Bundle("Core"=w221, "Your Boolean data"=w223, "Your string data"=w222) -> (w225:T5)  [unwired: 1 in]
        n71 = call <vilib>:"Add State(s) to Queue__JKI_lib_State_Machine.vi"("State(s) in (\"\")"=w227) -> ("States Out"=w226:string)  [unwired: 14 in]
      }
      frame "Data: Cleanup" {
        # "Cleanup any data and references, here.\n(this is called automatically, by the Macro: Exit)"
        n72 = Unbundle By Name(w229) -> ("Core.Current VI Reference"=w232:refnum<vi>)
        n73 = Close Reference(reference=w232, error in (no error)=w231) -> (error out=w230:errorcluster)
        n74 = call <vilib>:"Add State(s) to Queue__JKI_lib_State_Machine.vi"("State(s) in (\"\")"=w234) -> ("States Out"=w233:string)  [unwired: 14 in]
      }
      frame "---------- Events ----------" {
        # "Do not put any code in this frame.\n(It is a separator no-op. You can make a copy of this frame to create a new UI frame)"
        n75 = call <vilib>:"Add State(s) to Queue__JKI_lib_State_Machine.vi"("State(s) in (\"\")"=w239) -> ("States Out"=w238:string)  [unwired: 14 in]
      }
      frame "Events: Register" {
        # "Register message event to break Waiting in Event structure."
        n76 = call "CSM - Get New State Notifier Event.vi"("Name (\"\" to Use UUID) In"=w242) -> ("error out"=w240:errorcluster, "New State Notifier Event"=w241:refnum<user-event>)  [unwired: 9 in]
        n77 = register-events(w241) -> (reference out=w243:refnum<event-registration>)  [unwired: 2 in, 1 out]
      }
      frame "Events: Unregister" {
        n78 = Unregister For Events(event registration refnum=w246, error in=w250) -> (error out=w247:errorcluster)
      }
      frame "---------- UI ----------" {
        # "Do not put any code in this frame.\n(It is a separator no-op. You can make a copy of this frame to create a new UI frame)"
        n79 = call <vilib>:"Add State(s) to Queue__JKI_lib_State_Machine.vi"("State(s) in (\"\")"=w255) -> ("States Out"=w254:string)  [unwired: 14 in]
      }
      frame "UI: Initialize" {
        # "Initialize the User Interface, here.\n(this is called automatically, by the Macro: Init)"
        n80 = call <vilib>:"Add State(s) to Queue__JKI_lib_State_Machine.vi"("State(s) in (\"\")"=w260) -> ("States Out"=w259:string)  [unwired: 14 in]
      }
      frame "UI: Cursor Set" {
        # "Argument"
        # "Set and Unset Cursor Busy.\n(Usage: \"UI: Cursor Set >> Busy|Idle\")"
        n81 = case shown="\"Idle\", Default" w262 {
          tunnel: w264 -> [w269 w271]
          tunnel: [w268 w270] -> w263
          frame "Idle", Default {
            n82 = call <vilib>:"Unset Busy.vi"("error in (no error)"=w269) -> ("error out"=w268:errorcluster)  [unwired: 10 in]
          }
          frame "Busy" {
            n83 = call <vilib>:"Set Busy.vi"("error in (no error)"=w271) -> ("error out"=w270:errorcluster)  [unwired: 9 in, 1 out]
          }
        }
        n84 = call <vilib>:"Add State(s) to Queue__JKI_lib_State_Machine.vi"("State(s) in (\"\")"=w267) -> ("States Out"=w266:string)  [unwired: 14 in]
      }
      frame "UI: Front Panel State" {
        # "Argument"
        # "Set Front Panel Open or Closed\n(Usage: \"UI: Front Panel State >> Open|Close\")"
        n85 = Unbundle By Name(w275) -> ("Core.Current VI Reference"=w274:refnum<vi>)
        n86 = call <vilib>:"Add State(s) to Queue__JKI_lib_State_Machine.vi"("State(s) in (\"\")"=w279) -> ("States Out"=w278:string)  [unwired: 14 in]
        n87 = case shown="\"Minimize\", \"Minimized\"" w273 {
          tunnel: w277 -> [w285 w300 w311 w324 w337]
          tunnel: [w287 w301 w313 w326 w339] -> w276
          tunnel: w274 -> [w286 w298 w312 w325 w338]
          frame "Open", "Standard", Default {
            w280 = T1."Standard" ("State")
            n88 = property class="VI"(reference=w286, error in=w285) -> (reference out=w283:refnum<vi>, error out=w284:errorcluster, "FP.State"=w282:T1)
            n89 = Not Equal?(x=w282, y=w280) -> (x != y?=w281:bool)
            n90 = case shown="True" w281 {
              tunnel: [w291 w293] -> w287
              tunnel: w284 -> [w290 w293]
              tunnel: w283 -> [w289 _]
              tunnel: w280 -> [w288 _]
              frame True {
                n91 = invoke class="VI" method="FP.Open"(reference=w289, error in=w290, "Activate"=TRUE, "State"=w288) -> (error out=w291:errorcluster)  [unwired: 1 in, 4 out]
              }
              frame False {
              }
            }
          }
          frame "Close", "Closed" {
            n92 = property class="VI"(reference=w298, error in=w300) -> (reference out=w297:refnum<vi>, error out=w299:errorcluster, "FP.State"=w295:T1)
            n93 = Not Equal?(x=w295, y=T1."Closed" ("Front Panel Window:State")) -> (x != y?=w294:bool)
            n94 = case shown="True" w294 {
              tunnel: [w302 w305] -> w301
              tunnel: w299 -> [w302 w304]
              tunnel: w297 -> [_ w303]
              frame False {
              }
              frame True {
                n95 = invoke class="VI" method="FP.Close"(reference=w303, error in=w304) -> (error out=w305:errorcluster)  [unwired: 1 in, 2 out]
              }
            }
          }
          frame "Hidden", "Hide" {
            w306 = T1."Hidden" ("State")
            n96 = property class="VI"(reference=w312, error in=w311) -> (reference out=w309:refnum<vi>, error out=w310:errorcluster, "FP.State"=w308:T1)
            n97 = Not Equal?(x=w308, y=w306) -> (x != y?=w307:bool)
            n98 = case shown="True" w307 {
              tunnel: [w317 w318] -> w313
              tunnel: w310 -> [w316 w318]
              tunnel: w309 -> [w315 _]
              tunnel: w306 -> [w314 _]
              frame True {
                n99 = invoke class="VI" method="FP.Open"(reference=w315, error in=w316, "State"=w314) -> (error out=w317:errorcluster)  [unwired: 2 in, 4 out]
              }
              frame False {
              }
            }
          }
          frame "Minimize", "Minimized" {
            w319 = T1."Minimized" ("State")
            n100 = property class="VI"(reference=w325, error in=w324) -> (reference out=w322:refnum<vi>, error out=w323:errorcluster, "FP.State"=w321:T1)
            n101 = Not Equal?(x=w321, y=w319) -> (x != y?=w320:bool)
            n102 = case shown="True" w320 {
              tunnel: [w330 w331] -> w326
              tunnel: w323 -> [w329 w331]
              tunnel: w322 -> [w328 _]
              tunnel: w319 -> [w327 _]
              frame True {
                n103 = invoke class="VI" method="FP.Open"(reference=w328, error in=w329, "State"=w327) -> (error out=w330:errorcluster)  [unwired: 2 in, 4 out]
              }
              frame False {
              }
            }
          }
          frame "Maximize", "Maximized" {
            w332 = T1."Maximized" ("State")
            n104 = property class="VI"(reference=w338, error in=w337) -> (reference out=w335:refnum<vi>, error out=w336:errorcluster, "FP.State"=w334:T1)
            n105 = Not Equal?(x=w334, y=w332) -> (x != y?=w333:bool)
            n106 = case shown="True" w333 {
              tunnel: [w343 w344] -> w339
              tunnel: w336 -> [w342 w344]
              tunnel: w335 -> [w341 _]
              tunnel: w332 -> [w340 _]
              frame True {
                n107 = invoke class="VI" method="FP.Open"(reference=w341, error in=w342, "State"=w340) -> (error out=w343:errorcluster)  [unwired: 2 in, 4 out]
              }
              frame False {
              }
            }
          }
        }
      }
      frame "---------- Macro ----------" {
        # "Do not put any code in this frame.\n(It is a separator no-op. You can make a copy of this frame to create a new Macro frame)"
        n108 = call <vilib>:"Add State(s) to Queue__JKI_lib_State_Machine.vi"("State(s) in (\"\")"=w349) -> ("States Out"=w348:string)  [unwired: 14 in]
      }
      frame "Macro: Initialize" {
        w351 = "Data: Initialize\nInitialize Core Data\nEvents: Register\nUI: Initialize\nUI: Front Panel State >> Open\nMacro: Switch Active Module"  # Data: Initialize Initialize Core Data Events: Register UI: Initialize UI: Front Panel State >> Open Macro: Switch Active Module
        # "Initialization Macro\n(This is called once, when the VI starts)"
        n109 = call <vilib>:"Add State(s) to Queue__JKI_lib_State_Machine.vi"("State(s) in Front (\"\")"=w351, "State(s) in (\"\")"=w355) -> ("States Out"=w354:string)  [unwired: 13 in]
      }
      frame "Macro: Switch Active Module" {
        # "For Sync message, if the module name is fixed, you can use\nString constance with content \"API: Get Level -@ modulename\" instead of the helper VI."
        n110 = call-poly "Build Message with Arguments++.vi"("State With Arguments"="API: Get Level" ("State(s) in Front (\"\")"), "Target Module (\"\")"="SubModule" ("Name(\"\" to use uuid)")) -> ("CSM Message String"=w357:string)  [unwired: 13 in]
        n111 = call <vilib>:"Add State(s) to Queue__JKI_lib_State_Machine.vi"("State(s) in Front (\"\")"=w357, "State(s) in (\"\")"=w360) -> ("States Out"=w361:string)  [unwired: 13 in]
      }
      frame "Macro: Exit" {
        # "Exit Macro\n(This is called once, when the VI exits)"
        n112 = Unbundle By Name(w375) -> ("Core.Close Panel on Exit?"=w374:bool)
        n113 = call "CSM - Module Status.vi"("CSM Name"="SubModule") -> ("#Instance"=w366:i32)  [unwired: 6 in, 4 out]
        n114 = for {
          N: w366 -> [_]
          tunnel: ["Macro: Exit -@SubModule" ("CSM Name")] -> w365 mode=indexing
        }
        n115 = Select(t="UI: Front Panel State >> Close", s=w374, f="") -> (s? t:f=w371:string)
        n116 = call "CSM - Compact Multiple States.vi"("Multiple States"=w365) -> ("States"=w364:string)  [unwired: 9 in]
        n117 = call <vilib>:"Add State(s) to Queue__JKI_lib_State_Machine.vi"("State(s) in Front (\"\")"=w364, "State(s) in (\"\")"=w371, "State(s) at Back (\"\")"="Data: Cleanup\nEvents: Unregister\nExit") -> ("States Out"=w369:string)  [unwired: 12 in]
        n118 = call <vilib>:"Add State(s) to Queue__JKI_lib_State_Machine.vi"("State(s) in Front (\"\")"=w369, "State(s) in (\"\")"=w378) -> ("States Out"=w377:string)  [unwired: 13 in]
      }
      frame "------- Action -------" {
      }
      frame "Action: Status Chanage Handler" {
        # "No Code here. \nBut you can see the log when it's called because of the registered status change."
      }
    }
  }
  n119 = call "CSM - Mark As Worker Module.vi"("CSM Name"="SubModule" ("Name(\"\" to use uuid)")) -> ("CSM Name (Marked As Worker)"=w1:string)  [unwired: 9 in]
  n120 = call "CSM Reuse Module.vi"("Name (\"\" to Use UUID)"=w1) -> ()  [unwired: 11 in]
  n121 = call "CSM Reuse Module.vi"("Name (\"\" to Use UUID)"=w1) -> ()  [unwired: 11 in]
  n122 = call "CSM Reuse Module.vi"("Name (\"\" to Use UUID)"=w1) -> ()  [unwired: 11 in]
  n123 = call "CSM Reuse Module.vi"("Name (\"\" to Use UUID)"=w1) -> ()  [unwired: 11 in]
